vi "Ask Controller to Launch Results UI.vi"(8 "error in (no error)":errorcluster, 11 "Operator UI in":refnum<class "Measurement UI.lvclass">) -> (0 "error out":errorcluster, 3 "Operator UI out":refnum<class "Measurement UI.lvclass">)   [LabVIEW 2015, in "Measurement UI.lvlib" / "Measurement UI.lvclass"]
uses:
  Measurement UI.lvclass
  Measurement UI.lvclass/Measurement UI.ctl
  <vilib>/ActorFramework/Actor/Actor.lvclass/Actor.ctl
  Controller/Messages/Launch Results UI Msg/Launch Results UI Msg.lvclass/Launch Results UI Msg.ctl
  <vilib>/ActorFramework/Message Enqueuer/Message Enqueuer.lvclass/Message Enqueuer.ctl
  Accessors/Read Results Listbox.vi
  <vilib>/ActorFramework/Message Enqueuer/Enqueue.vi
  <vilib>/ActorFramework/Message Priority Queue/Priority Enqueue.vi
  Controller/Messages/Launch Results UI Msg/Launch Results UI Msg.lvclass
  User Interface/UI.lvclass
  <vilib>/ActorFramework/Actor/Actor.lvclass
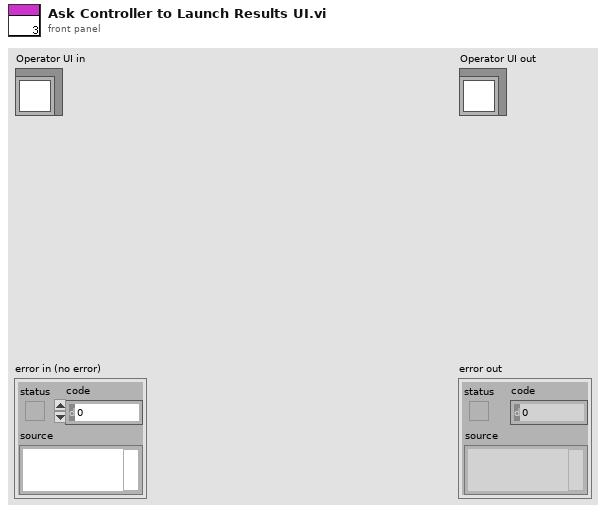
[diagram p1: front panel]
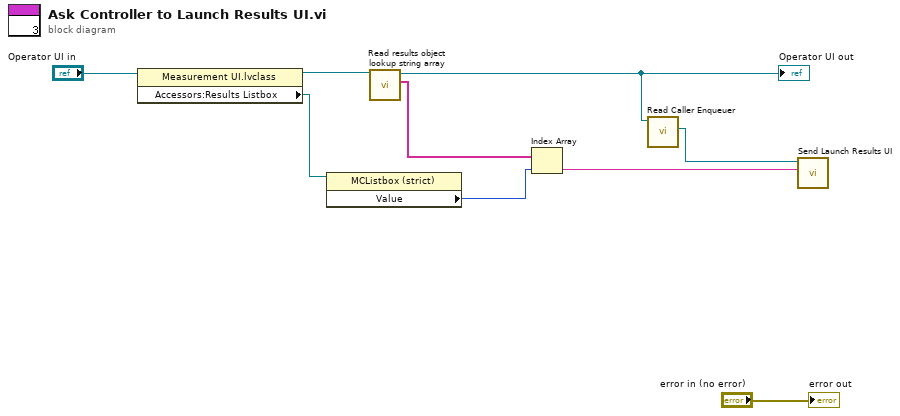
[diagram p0: block diagram]
diagram:
  n1 = property class="Measurement UI.lvclass"(reference="Operator UI in") -> (reference out=w1:refnum<class "Measurement UI.lvclass">, "Accessors:Results Listbox"=w2:refnum<vi>)  [unwired: 1 in, 1 out]
  n2 = property class="MCListbox (strict)"(reference=w2) -> ("Value"=w8:i32)  [unwired: 1 in, 2 out]
  n3 = call "Read results object lookup string array.vi"("UI in"=w1) -> ("results object lookup string array"=w7:string[], "UI out"=w5:refnum<class "Measurement UI.lvclass">)  [unwired: 8 in, 1 out]
  "Operator UI out" <- w5
  n4 = Index Array(array=w7, index=w8) -> (element=w6:string)
  n5 = call <vilib>:"Read Caller Enqueuer.vi"("Actor"=w5) -> ("Caller Enqueuer"=w4:refnum<class "Message Enqueuer.lvclass">)  [unwired: 10 in]
  n6 = call "Send Launch Results UI.vi"("uniqueresultsid"=w6, "Message Enqueuer in"=w4) -> ()  [unwired: 8 in, 2 out]
  "error out" <- "error in (no error)"
